vi "质控参数保存.vi"(7 "section":string="氨氮质控参数", 8 "error in (no error)":errorcluster caption="错误输入（无错误）", 11 "参数":T1) -> (0 "error out":errorcluster caption="错误输出")   [LabVIEW 2016, in "质控单元.lvlib"]
uses:
  <vilib>/Utility/config.llb/Write Key (Double).vi
  <vilib>/Utility/config.llb/NI_LVConfig.lvlib
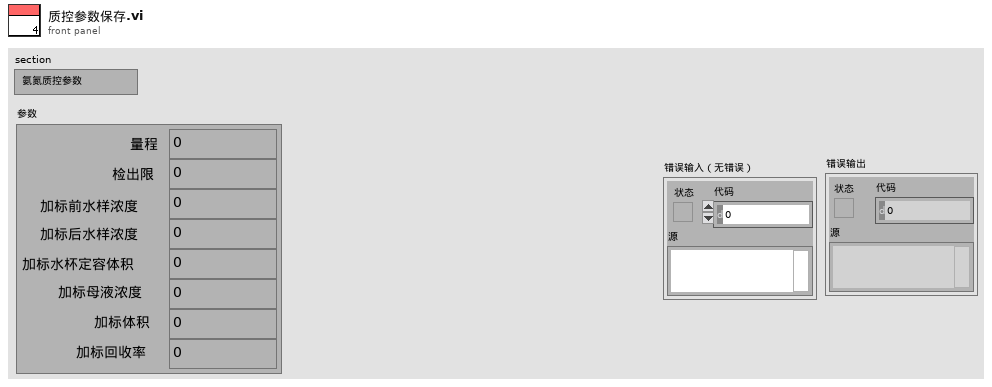
[diagram p1: front panel]
types:
  T1 = cluster{"量程":dbl, "检出限":dbl, "加标前水样浓度":dbl, "加标后水样浓度":dbl, "加标水杯定容体积":dbl, "加标母液浓度":dbl, "加标体积":dbl, "加标回收率":dbl}
  T2 = typedef "NI_LVConfig.lvlib/Config Data RefNum.ctl" = refnum<k1>
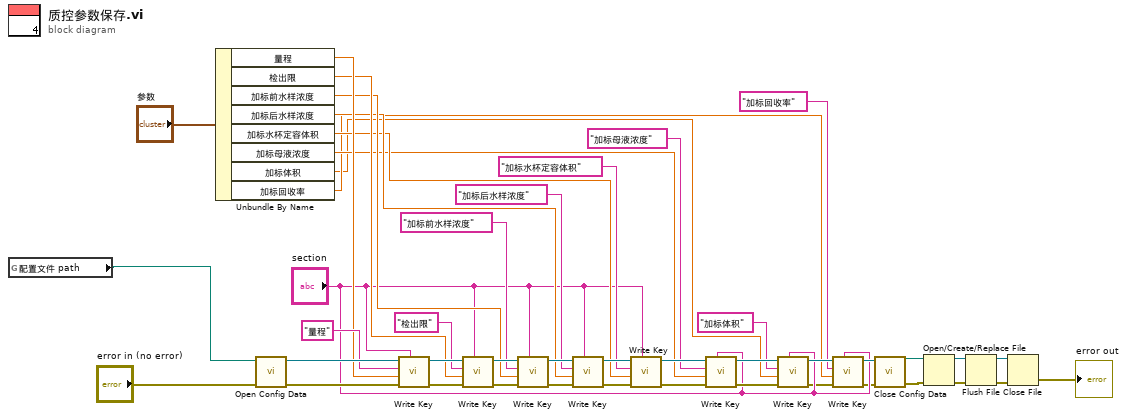
[diagram p0: block diagram]
diagram:
  n1 = global read "质控内部交互全局.vi" "配置文件 path"() -> (w1:path)
  n2 = Unbundle By Name("参数") -> ("量程"=w25:dbl, "检出限"=w24:dbl, "加标前水样浓度"=w23:dbl, "加标后水样浓度"=w22:dbl, "加标水杯定容体积"=w21:dbl, "加标母液浓度"=w20:dbl, "加标体积"=w9:dbl, "加标回收率"=w10:dbl)
  n3 = call <vilib>:"Open Config Data.vi"("error in (no error)"="error in (no error)", "configuration file path"=w1) -> ("error out"=w44:errorcluster, "refnum"=w45:T2)  [unwired: 7 in, 1 out]
  n4 = call-poly <vilib>:"Write Key.vi"("section"="section", "error in (no error)"=w44, "value"=w25, "key"="量程", "refnum"=w45) -> ("error out"=w41:errorcluster, "refnum out"=w42:T2)  [unwired: 4 in, 1 out]
  n5 = call-poly <vilib>:"Write Key.vi"("section"="section", "error in (no error)"=w41, "value"=w24, "key"="检出限", "refnum"=w42) -> ("error out"=w39:errorcluster, "refnum out"=w40:T2)  [unwired: 4 in, 1 out]
  n6 = call-poly <vilib>:"Write Key.vi"("section"="section", "error in (no error)"=w39, "value"=w23, "key"="加标前水样浓度", "refnum"=w40) -> ("error out"=w33:errorcluster, "refnum out"=w34:T2)  [unwired: 4 in, 1 out]
  n7 = call-poly <vilib>:"Write Key.vi"("section"="section", "error in (no error)"=w33, "value"=w22, "key"="加标后水样浓度", "refnum"=w34) -> ("error out"=w36:errorcluster, "refnum out"=w35:T2)  [unwired: 4 in, 1 out]
  n8 = call-poly <vilib>:"Write Key.vi"("section"="section", "error in (no error)"=w36, "value"=w21, "key"="加标水杯定容体积", "refnum"=w35) -> ("error out"=w38:errorcluster, "refnum out"=w37:T2)  [unwired: 4 in, 1 out]
  n9 = call-poly <vilib>:"Write Key.vi"("section"="section", "error in (no error)"=w38, "value"=w20, "key"="加标母液浓度", "refnum"=w37) -> ("error out"=w19:errorcluster, "refnum out"=w18:T2)  [unwired: 4 in, 1 out]
  n10 = call-poly <vilib>:"Write Key.vi"("section"="section", "error in (no error)"=w19, "value"=w9, "key"="加标体积", "refnum"=w18) -> ("error out"=w12:errorcluster, "refnum out"=w17:T2)  [unwired: 4 in, 1 out]
  n11 = call-poly <vilib>:"Write Key.vi"("section"="section", "error in (no error)"=w12, "value"=w10, "key"="加标回收率", "refnum"=w17) -> ("error out"=w11:errorcluster, "refnum out"=w16:T2)  [unwired: 4 in, 1 out]
  n12 = call <vilib>:"Close Config Data.vi"("error in (no error)"=w11, "refnum"=w16) -> ("error out"=w4:errorcluster, "file path"=w3:path)  [unwired: 8 in]
  n13 = Open/Create/Replace File(file path (use dialog)=w3, error in=w4) -> (refnum out=w6:refnum<file>, error out=w5:errorcluster)  [unwired: 4 in, 1 out]
  n14 = Flush File(refnum=w6, error in=w5) -> (refnum out=w7:refnum<file>, error out=w8:errorcluster)
  n15 = Close File(refnum=w7, error in=w8) -> (error out=→"error out":errorcluster)  [unwired: 1 out]
